vi "SetMeasureFilterType.vi"(7 "SMU":T1, 8 "Error In":errorcluster, 10 "Filter Type":T2, 11 "Keithley 2602 In":refnum<visa-resource-name>) -> (0 "Error Out":errorcluster, 3 "Keithley 2602 Out":refnum<visa-resource-name>)   [LabVIEW 2012, in "Keithley-2602.lvlib"]
uses:
  Keithley-2602.lvlib
  Controls/FilterType.ctl
  Controls/SMU.ctl
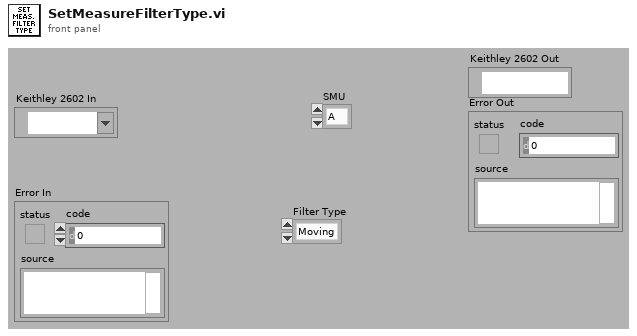
[diagram p1: front panel]
types:
  T1 = typedef "Keithley-2602.lvlib/SMU.ctl" = enum16{"A", "B"}
  T2 = typedef "Keithley-2602.lvlib/FilterType.ctl" = enum16{"Moving", "Repeating", "Median"}
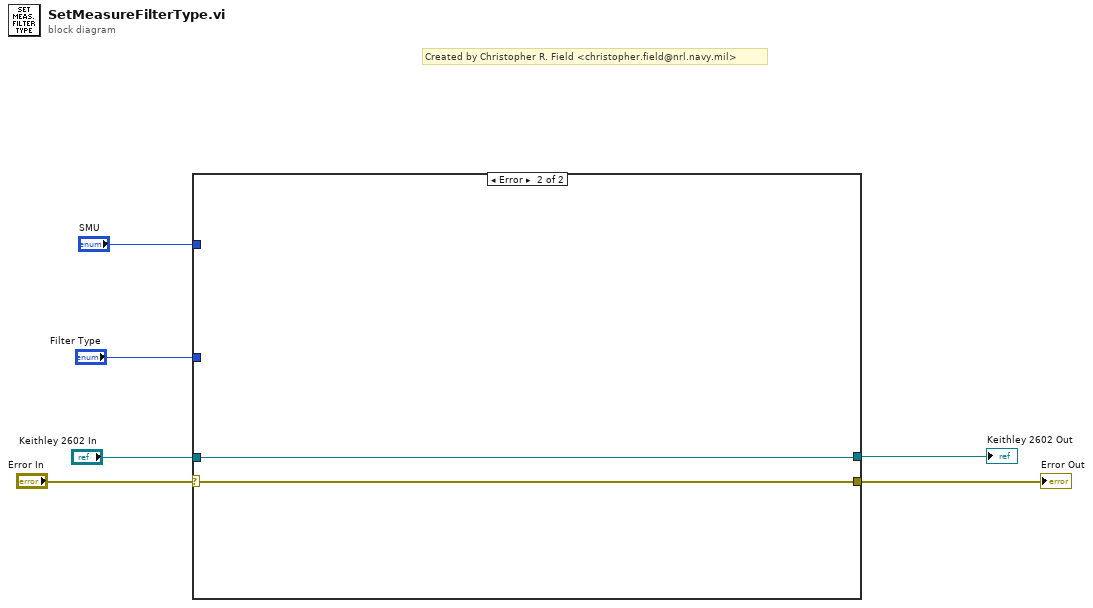
[diagram p0: block diagram]
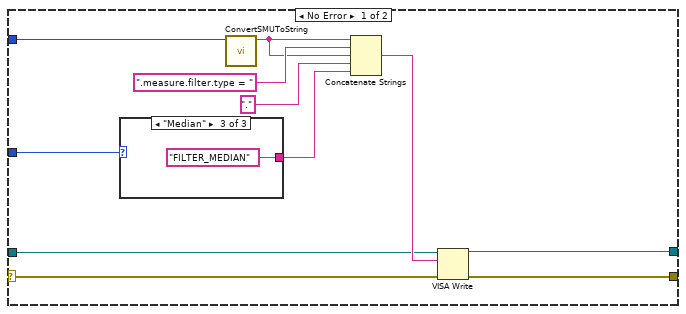
[diagram p2: hidden frame]
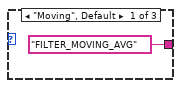
[diagram p3: hidden frame]
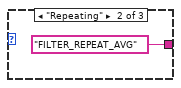
[diagram p4: hidden frame]
diagram:
  # "Created by Christopher R. Field <christopher.field@nrl.navy.mil>"
  n1 = case shown="Error" "Error In" {
    selector: "Error In" -> [w7 w21]
    tunnel: "Keithley 2602 In" -> [w12 w22]
    tunnel: [w11 w22] -> w5
    tunnel: [w10 w21] -> w4
    tunnel: "SMU" -> [w9 _]
    tunnel: "Filter Type" -> [w8 _]
    frame No Error {
      n2 = case shown="\"Median\"" w8 {
        tunnel: ["FILTER_MOVING_AVG" "FILTER_REPEAT_AVG" "FILTER_MEDIAN"] -> w14
        frame "Moving", Default {
        }
        frame "Repeating" {
        }
        frame "Median" {
        }
      }
      n3 = call "ConvertSMUToString.vi"("SMU"=w9) -> ("Channel"=w16:string)  [unwired: 10 in]
      n4 = Concatenate Strings(w16, ".measure.filter.type = ", w16, "." ("string"), w14) -> (w13:string)
      n5 = VISA Write(VISA resource name=w12, write buffer=w13, error in (no error)=w7) -> (VISA resource name out=w11:refnum<visa-resource-name>, error out=w10:errorcluster)  [unwired: 1 out]
    }
    frame Error {
    }
  }
  "Keithley 2602 Out" <- w5
  "Error Out" <- w4
